vi "Generate Tree from 2D array.vi"(8 "error in (no error)":errorcluster, 10 "XML 2D Array":string[][](array[string])=[["OME", "xsi:schemaLocation", "http://www.openmicroscopy.org/Schemas/OME/2015-01                         http://www.openmicroscopy.org/Schemas/OME/2015-01/ome.xsd", "", "", "", ""], ["OME", "Experiment", "ID", "2PExperiment", "", "", ""], ["OME", "Experiment", "Description", "Description", "XYZ behavioral study", "", ""], ["OME", "Experiment", "ExperimenterRef", "ID", "Experimenter001", "", ""], ["OME", "Experimenter", "Email", "abc@xyz.com", "", "", ""], ["OME", "Experimenter", "FirstName", "FirstName", "", "", ""], ["OME", "Experimenter", "ID", "Experimenter001", "", "", ""], ["OME", "Experimenter", "Institution", "*", "", "", ""], ["OME", "Experimenter", "LastName", "LastName", "", "", ""], ["OME", "File", "Format", "*", "", "", ""], ["OME", "File", "ID", "*", "", "", ""], ["OME", "File", "Name", "*", "", "", ""], ["OME", "File", "absPath", "*", "", "", ""], ["OME", "File", "relPath", "*", "", "", ""], ["OME", "File", "rootPath", "*", "", "", ""], ["OME", "Sample", "Age", "*", "", "", ""], ["OME", "Sample", "Description", "*", "", "", ""], ["OME", "Sample", "ID", "*", "", "", ""], ["OME", "Instrument", "ID", "Instrument:0", "", "", ""], ["OME", "Instrument", "Microscope", "Manufacturer", "Scientifica", "", ""], ["OME", "Instrument", "Microscope", "Model", "MP1000", "", ""], ["OME", "Instrument", "Microscope", "SoftwareVersion", "d", "", ""], ["OME", "Instrument", "LightSource", "ID", "*", "", ""], ["OME", "Instrument", "LightSource", "Laser", "LaserMedium", "TiSapphire", ""], ["OME", "Instrument", "LightSource", "Laser", "Type", "SolidState", ""], ["OME", "Instrument", "LightSource", "SerialNo", "f", "", ""], ["OME", "Instrument", "Detector", "ID", "Detector:0:0", "", ""], ["OME", "Instrument", "Detector", "Manufacturer", "Hamamatzu", "", ""], ["OME", "Instrument", "Detector", "Model", "xxxxxx", "", ""], ["OME", "Instrument", "Detector", "Type", "PMT (Multialkali)", "", ""], ["OME", "Instrument", "Detector", "ID", "Detector:0:1", "", ""], ["OME", "Instrument", "Detector", "Manufacturer", "New Manufacturer", "", ""], ["OME", "Instrument", "Detector", "Model", "yyyyyy", "", ""], ["OME", "Instrument", "Detector", "Type", "PMT (GaAsP)", "", ""], ["OME", "Instrument", "Objective", "ID", "Objective:10002", "", ""], ["OME", "Instrument", "Objective", "Immersion", "Water", "", ""], ["OME", "Instrument", "Objective", "LensNA", "1.4", "", ""], ["OME", "Instrument", "Objective", "Manufacturer", "Olympus", "", ""], ["OME", "Instrument", "Objective", "NominalMagnification", "100", "", ""], ["OME", "Image", "ID", "Default", "", "", ""], ["OME", "Image", "Name", "Default", "", "", ""], ["OME", "Image", "AcquisitionDate", "AcquisitionDate", "2011-09-16T10:45:48", "", ""], ["OME", "Image", "Description", "Description", " OME compatible file ", "", ""], ["OME", "Image", "Pixels", "DimensionOrder", "XYCZT", "", ""], ["OME", "Image", "Pixels", "ID", "Pixels:0", "", ""], ["OME", "Image", "Pixels", "SizeC", "1", "", ""], ["OME", "Image", "Pixels", "Channel", "DetectorSettings", "Binning", "1x1"], ["OME", "Image", "Pixels", "Channel", "DetectorSettings", "Gain", "0.5"], ["OME", "Image", "Pixels", "Channel", "DetectorSettings", "ID", "Detector:0:0"], ["OME", "Image", "Pixels", "Channel", "DetectorSettings", "ReadOutRate", "10.0"], ["OME", "Image", "Pixels", "Type", "int8", "", ""], ["OME", "Image", "Pixels", "Channel", "ID", "Channel:1:2", ""], ["OME", "Image", "Pixels", "Channel", "IlluminationType", "Epifluorescence", ""], ["OME", "Image", "Pixels", "Channel", "NDFilter", "0.0", ""], ["OME", "Image", "Pixels", "Channel", "Name", "RD-TR-PE", ""], ["OME", "Image", "Pixels", "Channel", "SamplesPerPixel", "1", ""]], 11 "Tree Refnum":refnum<vi>) -> (0 "error out":errorcluster)   [LabVIEW 2012]
doc: "SciScan 1.2 160622"
panel:
  out "Array":i32[](array[numeric])
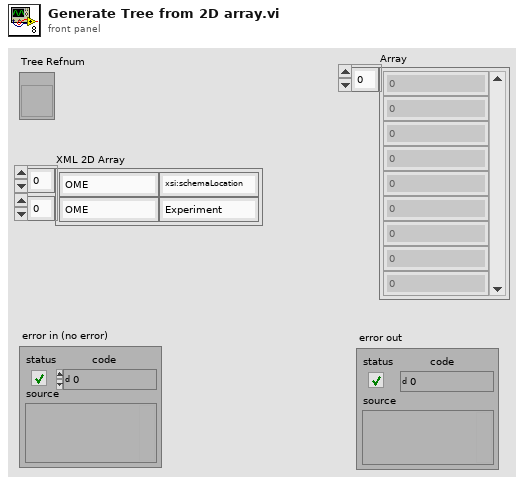
[diagram p1: front panel]
types:
  T1 = cluster{"Left Cell String":string, "Child Text":string[], "Child Tag":string, "Item Indent":i32, "Child Only?":bool, "Glyph Index":i32}
  T2 = cluster{"Left Cell String":string, "Child Text":string[], "Child Tag":string, "Item Indent":i32, "Child Only?":bool, "Glyph Index":i32}[]
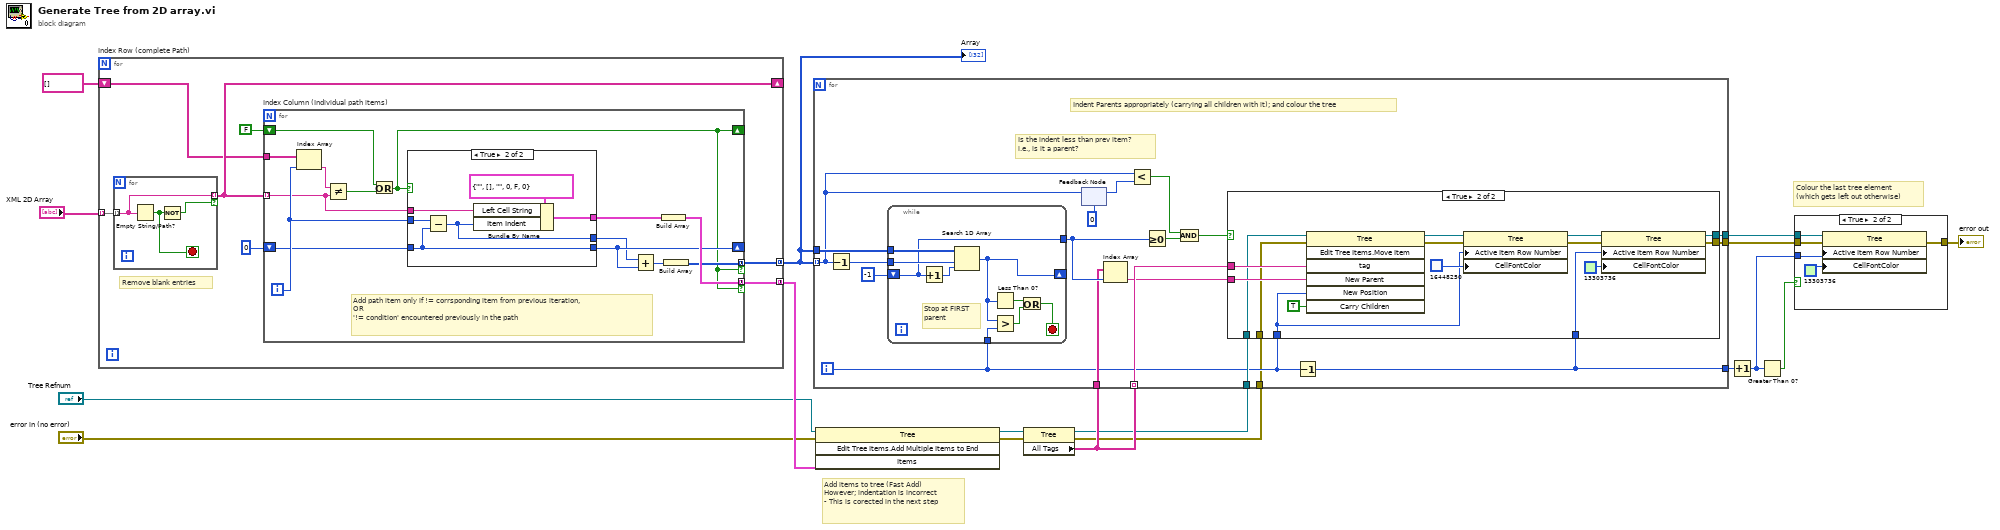
[diagram p0: block diagram]
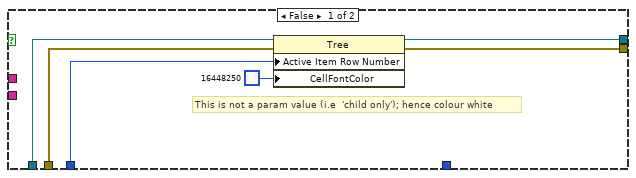
[diagram p3: hidden frame]
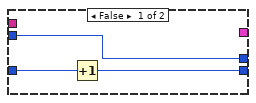
[diagram p4: hidden frame]
diagram:
  # "Colour the last tree element\n(which gets left out otherwise)"
  # "Add items to tree (Fast Add)\nHowever; indentation is incorrect\n- This is corected in the next step"
  n1 = for "Index Row (complete Path)" {
    tunnel: "XML 2D Array" -> [w23] mode=indexing
    tunnel: [w24] -> w17 mode=concatenating
    shift-right: [w22] -> _
    shift-left: string[] [] -> [w21]
    tunnel: [w19] -> w12 mode=concatenating
    # "Remove blank entries"
    n2 = for {
      tunnel: w23 -> [w50] mode=indexing
      tunnel: [w50] -> w22 mode=indexing if=w48
      stop <- w49 stop-if-true
      n3 = Empty String/Path?(string/path=w50) -> (empty?=w49:bool)
      n4 = Not(x=w49) -> (.not. x?=w48:bool)
    }
    n5 = for "Index Column (Individual path items)" {
      tunnel: [w37] -> w24 mode=concatenating if=w29
      tunnel: w22 -> [w33] mode=indexing
      tunnel: w21 -> [w36]
      shift-right: [w30] -> _
      shift-left: 0 -> [w32]
      tunnel: [w31] -> w19 mode=concatenating if=w29
      shift-right: [w29] -> _
      shift-left: FALSE -> [w28]
      i -> [w35]
      # "Add path item only if != corrsponding item from previous iteration,\nOR\n'!= condition' encountered previously in the path"
      n6 = Index Array(array=w36, index=w35) -> (element=w34:string)
      n7 = Not Equal?(x=w34, y=w33) -> (x != y?=w25:bool)
      n8 = Or(x=w28, y=w25) -> (x .or. y?=w29:bool)
      n9 = case shown="True" w29 {
        tunnel: [_ w47] -> w38
        tunnel: w33 -> [_ w46]
        tunnel: w35 -> [w39 w44]
        tunnel: [w40 w45] -> w30
        tunnel: w32 -> [w41 w45]
        tunnel: [w39 w43] -> w26
        frame False {
          n10 = Increment(x=w41) -> (x+1=w40:i32)
        }
        frame True {
          n11 = Subtract(x=w44, y=w45) -> (x-y=w43:i32)
          n12 = Bundle By Name(cluster=T1 {"Left Cell String"="", "Child Text"=[], "Child Tag"="", "Item Indent"=0, "Child Only?"=FALSE, "Glyph Index"=0} ("Item"), "Left Cell String"=w46, "Item Indent"=w43) -> (w47:T1)
        }
      }
      n13 = Add(x=w26, y=w30) -> (x+y=w27:i32)
      n14 = Build Array(w38) -> (w37:T2)
      n15 = Build Array(w27) -> (w31:i32[])
    }
  }
  "Array" <- w12
  n16 = invoke class="Tree" method="Edit Tree Items.Add Multiple Items to End"(reference="Tree Refnum", error in="error in (no error)", "Items"=w17) -> (reference out=w15:refnum<vi>, error out=w11:errorcluster)  [unwired: 1 in, 2 out]
  n17 = property class="Tree"(reference=w15, error in=w11) -> (reference out=w13:refnum<vi>, error out=w10:errorcluster, "All Tags"=w14:string[])
  n18 = for {
    tunnel: w12 -> [w60] mode=indexing
    tunnel: w12 -> [w68]
    tunnel: w14 -> [w66] mode=indexing
    tunnel: w14 -> [w58]
    tunnel: w13 -> [w62]
    tunnel: w10 -> [w56]
    tunnel: [w55] -> w7
    tunnel: [w52] -> w6
    tunnel: [w51] -> w8
    i -> [w57]
    # "Is the indent less than prev item?\ni.e., is it a parent?"
    # "Indent Parents appropriately (carrying all children with it); and colour the tree"
    n19 = Decrement(x=w60) -> (x-1=w69:i32)
    n20 = while {
      tunnel: w69 -> [w99]
      tunnel: w68 -> [w98]
      shift-right: [w96] -> _
      shift-left: -1 ("index of element") -> [w91]
      tunnel: w57 -> [w97]
      tunnel: [w91] -> w64
      stop <- w92 stop-if-true
      # "Stop at FIRST\nparent"
      n21 = Increment(x=w91) -> (x+1=w95:i32)
      n22 = Search 1D Array(1D array=w98, element=w99, start index (0)=w95) -> (index of element=w96:i32)
      n23 = Less Than 0?(x=w96) -> (x < 0?=w94:bool)
      n24 = Greater?(x=w96, y=w97) -> (0:w93:bool)
      n25 = Or(x=w94, y=w93) -> (x .or. y?=w92:bool)
    }
    n26 = feedback #1(0) -> (w54:i32)
    n27 = feedback-in #1(w60) -> ()
    n28 = Index Array(array=w58, index=w64) -> (element=w65:string)
    n29 = Less?(x=w60, y=w54) -> (x < y?=w59:bool)
    n30 = Greater Or Equal To 0?(x=w64) -> (x >= 0?=w63:bool)
    n31 = And(x=w59, y=w63) -> (x .and. y?=w61:bool)
    n32 = Decrement(x=w57) -> (x-1=w52:i32)
    n33 = case shown="True" w61 {
      tunnel: w66 -> [_ w90]
      tunnel: w65 -> [_ w89]
      tunnel: w62 -> [w73 w88]
      tunnel: w57 -> [w74 w83]
      tunnel: w52 -> [_ w86]
      tunnel: w56 -> [w72 w79]
      tunnel: [w71 w78] -> w55
      tunnel: [w70 w77] -> w51
      frame False {
        # "This is not a param value (i.e  'child only'); hence colour white"
        n34 = property class="Tree"(reference=w73, error in=w72, "Active Item Row Number"=w74, "CellFontColor"=u32 16448250) -> (reference out=w70:refnum<vi>, error out=w71:errorcluster)
      }
      frame True {
        n35 = invoke class="Tree" method="Edit Tree Items.Move Item"(reference=w88, error in=w79, "tag"=w90, "New Parent"=w89, "New Position"=w83, "Carry Children"=TRUE ("Carry Children?")) -> (reference out=w84:refnum<vi>, error out=w81:errorcluster)  [unwired: 1 in, 5 out]
        n36 = property class="Tree"(reference=w84, error in=w81, "Active Item Row Number"=w83, "CellFontColor"=u32 16448250) -> (reference out=w82:refnum<vi>, error out=w80:errorcluster)
        n37 = property class="Tree"(reference=w82, error in=w80, "Active Item Row Number"=w86, "CellFontColor"=u32 13303736) -> (reference out=w77:refnum<vi>, error out=w78:errorcluster)
      }
    }
  }
  n38 = Increment(x=w6) -> (x+1=w5:i32)
  n39 = Greater Than 0?(x=w5) -> (x > 0?=w9:bool)
  n40 = case shown="True" w9 {
    tunnel: w5 -> [_ w104]
    tunnel: w8 -> [_ w103]
    tunnel: w7 -> [w100 w102]
    tunnel: [w100 w101] -> w3
    frame False {
    }
    frame True {
      n41 = property class="Tree"(reference=w103, error in=w102, "Active Item Row Number"=w104, "CellFontColor"=u32 13303736) -> (error out=w101:errorcluster)  [unwired: 1 out]
    }
  }
  "error out" <- w3
